vi "Demo.vi"() -> ()   [LabVIEW 2011]
uses:
  StatD Class/Controls/Event Types.ctl
  StatD Class/Controls/Priorities.ctl
  StatD Class/StatD Interface.lvclass
panel:
  in  "Priority (normal)":T1=enum."normal"
  in  "Aggregation Key":string
  in  "Send Event":bool
  in  "Event Type (info)":T2=enum."info"
  in  "Event Text":string
  in  "Event Title":string
  in  "stop":bool
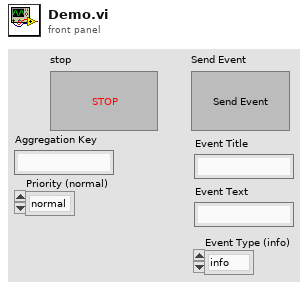
[diagram p1: front panel]
types:
  T1 = typedef "StatD Interface.lvclass/Priorities.ctl" = enum16{"low", "normal"}
  T2 = typedef "StatD Interface.lvclass/Event Types.ctl" = enum16{"error", "warning", "info", "success"}
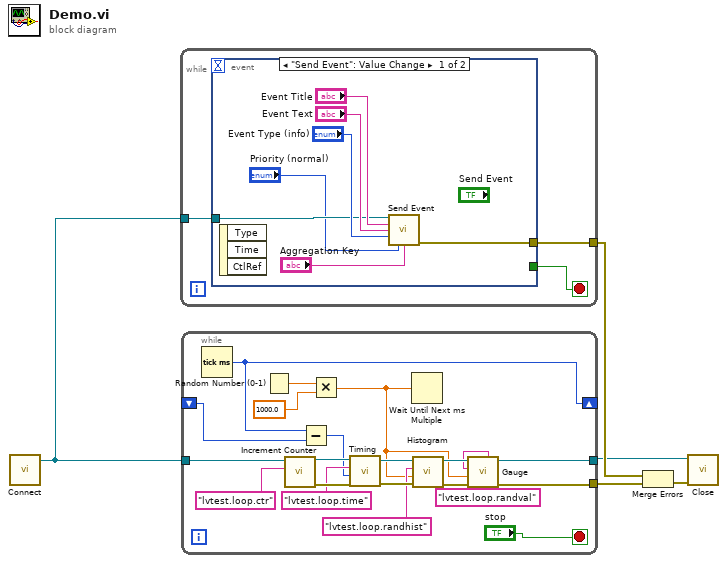
[diagram p0: block diagram]
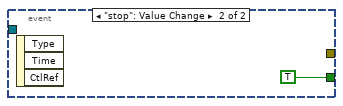
[diagram p2: hidden frame]
diagram:
  n1 = call "Connect.vi"() -> ("StatD Interface out"=w5:refnum<class "StatD Interface.lvclass">)  [unwired: 10 in, 1 out]
  n2 = while {
    tunnel: w5 -> [w7]
    tunnel: [w6] -> w4
    stop <- w8 stop-if-true
    n3 = event shown="[0] \"Send Event\": Value Change" {
      selector: _ -> [_ _]
      dyn-events: _ -> [_ _]
      timeout: _ -> [_ _]
      tunnel: [_ TRUE] -> w8
      tunnel: w7 -> [w12 _]
      tunnel: [w11 _] -> w6
      event "Send Event": Value Change {
        n4 = event-data() -> ()  [unwired: 1 in, 3 out]
        n5 = call "Send Event.vi"("StatD Interface in"=w12, "Event Title"="Event Title", "Event Text"="Event Text", "Event Type (info)"="Event Type (info)", "Priority (normal)"="Priority (normal)", "Aggregation Key (none)"="Aggregation Key") -> ("error out"=w11:errorcluster)  [unwired: 8 in, 1 out]
      }
      event "stop": Value Change {
        n6 = event-data() -> ()  [unwired: 1 in, 3 out]
      }
    }
  }
  n7 = while {
    tunnel: w5 -> [w33]
    shift-right: [w28] -> _
    shift-left: _ -> [w27]
    tunnel: [w18] -> w1
    tunnel: [w17] -> w3
    stop <- "stop" stop-if-true
    n8 = Tick Count (ms)() -> (millisecond timer value=w28:u32)
    n9 = Random Number (0-1)() -> (number: 0 to 1=w35:dbl)
    n10 = call "Increment Counter.vi"("Metric Name"="lvtest.loop.ctr", "StatD Interface in"=w33) -> ("error out"=w31:errorcluster, "StatD Interface out"=w30:refnum<class "StatD Interface.lvclass">)  [unwired: 8 in]
    n11 = Subtract(x=w28, y=w27) -> (x-y=w26:u32)
    n12 = Multiply(x=w35, y=1000.0) -> (x*y=w19:dbl)
    n13 = call "Timing.vi"("error in (no error)"=w31, "Time (ms)"=w26, "Metric Name"="lvtest.loop.time", "StatD Interface in"=w30) -> ("error out"=w24:errorcluster, "StatD Interface out"=w25:refnum<class "StatD Interface.lvclass">)  [unwired: 6 in]
    n14 = Wait Until Next ms Multiple(millisecond multiple=w19) -> ()  [unwired: 1 out]
    n15 = call "Histogram.vi"("error in (no error)"=w24, "Metric Value"=w19, "Metric Name"="lvtest.loop.randhist", "StatD Interface in"=w25) -> ("error out"=w22:errorcluster, "StatD Interface out"=w23:refnum<class "StatD Interface.lvclass">)  [unwired: 6 in]
    n16 = call "Gauge.vi"("error in (no error)"=w22, "Metric Value"=w19, "Metric Name"="lvtest.loop.randval", "StatD Interface in"=w23) -> ("error out"=w17:errorcluster, "StatD Interface out"=w18:refnum<class "StatD Interface.lvclass">)  [unwired: 6 in]
  }
  n17 = Merge Errors(w4, w3) -> (w2:errorcluster)
  n18 = call "Close.vi"("error in (no error)"=w2, "StatD Interface in"=w1) -> ()  [unwired: 9 in, 1 out]
